vi "DriveAtAngleForT.vi"(7 "time(sec)":dbl, 8 "Error In":errorcluster, 10 "y":dbl, 11 "x":dbl) -> (0 "Error Out":errorcluster)   [LabVIEW 2017]
panel:
  # "Drive at Angle for Time Autonomous Command\nFRC Team 34"
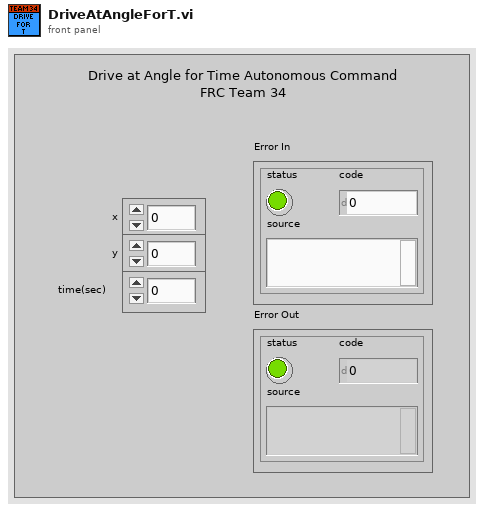
[diagram p1: front panel]
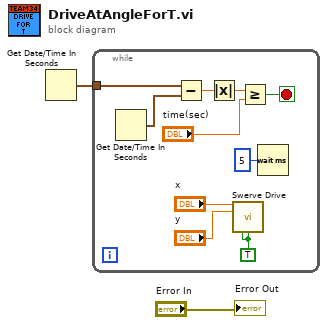
[diagram p0: block diagram]
diagram:
  n1 = Get Date/Time In Seconds() -> (seconds since 1Jan1904=w2:timestamp)
  n2 = while {
    tunnel: w2 -> [w12]
    stop <- w8 stop-if-true
    w3 = TRUE ("Autonomous?")
    n3 = Get Date/Time In Seconds() -> (seconds since 1Jan1904=w11:timestamp)
    n4 = Subtract(x=w12, y=w11) -> (x-y=w10:dbl)
    n5 = Absolute Value(x=w10) -> (abs(x)=w9:dbl)
    n6 = call "Swerve Drive.vi"("X"="x", "Y"="y", "Robot Centric?"=w3, "Autonomous?"=w3) -> ()  [unwired: 7 in, 5 out]
    n7 = Greater Or Equal?(x=w9, y="time(sec)") -> (x >= y?=w8:bool)
    n8 = Wait (ms)(milliseconds to wait=u32 5) -> ()  [unwired: 1 out]
  }
  "Error Out" <- "Error In"
